vi "ADIS16470 Scale Data.vi"(3 "TimeStamp":u32, 5 "Data In":u8[](array[numeric])) -> (1 "Data":T1)   [LabVIEW 2020]
uses:
  Typedef/ADIS16470 Data.ctl
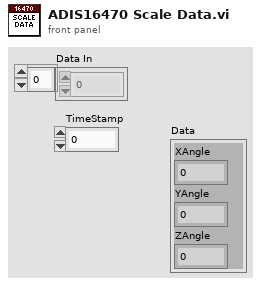
[diagram p1: front panel]
types:
  T1 = typedef "ADIS16470 Data.ctl" = cluster{"XAngle":dbl, "YAngle":dbl, "ZAngle":dbl}
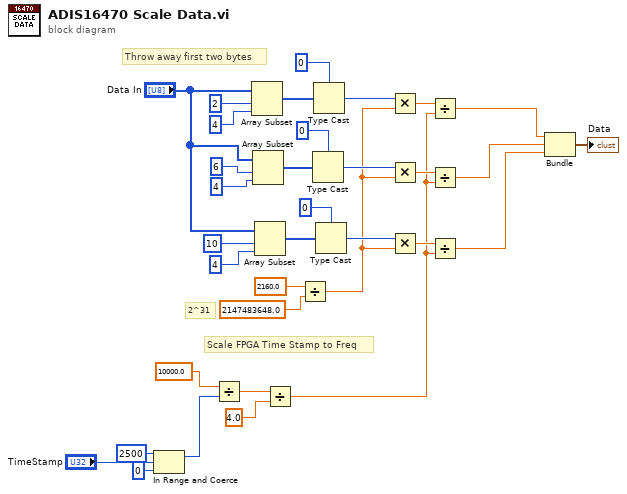
[diagram p0: block diagram]
diagram:
  # "Scale FPGA Time Stamp to Freq"
  # "2^31"
  # "Throw away first two bytes"
  n1 = In Range and Coerce(upper limit=u32 2500, x="TimeStamp", lower limit=u32 0) -> (coerced(x)=w1:u32)  [unwired: 1 out]
  n2 = Divide(x=10000.0, y=w1) -> (x/y=w11:dbl)
  n3 = Array Subset(array="Data In", index=2, length=4) -> (w27:u8[])
  n4 = Array Subset(array="Data In", index=6, length=4 ("index")) -> (w25:u8[])
  n5 = Array Subset(array="Data In", index=10, length=4) -> (w26:u8[])
  n6 = Divide(x=w11, y=4.0) -> (x/y=w9:dbl)
  n7 = Divide(x=2160.0, y=2147483648.0) -> (x/y=w16:dbl)
  n8 = Type Cast(type=0, x=w25) -> (*(type *) &x=w19:i32)
  n9 = Type Cast(type=0, x=w27) -> (*(type *) &x=w21:i32)
  n10 = Type Cast(type=0, x=w26) -> (*(type *) &x=w20:i32)
  n11 = Multiply(x=w21, y=w16) -> (x*y=w15:dbl)
  n12 = Multiply(x=w19, y=w16) -> (x*y=w14:dbl)
  n13 = Multiply(x=w20, y=w16) -> (x*y=w13:dbl)
  n14 = Divide(x=w15, y=w9) -> (x/y=w8:dbl)
  n15 = Divide(x=w14, y=w9) -> (x/y=w7:dbl)
  n16 = Divide(x=w13, y=w9) -> (x/y=w6:dbl)
  n17 = Bundle(w8, w7, w6) -> (→"Data":cluster{dbl, dbl, dbl})  [unwired: 1 in]
